vi "SV Change notification event builder.vi"(8 "error in (no error)":errorcluster, 11 "Guardian in":refnum<class "Guardian.lvclass">) -> (0 "error out":errorcluster, 3 "shared variable value change notification":refnum<user-event>)   [LabVIEW 2020, in "TALOS.lvlib" / "Guardian.lvlib" / "Guardian.lvclass"]
uses:
  Guardian.lvclass
  C:/Users/marco/Documents/GitHub_Lab/TALOS/talos/Ancestor/Ancestor/Ancestor.lvclass
  Ancestor/Ancestor/Ancestor.lvclass/Ancestor.ctl
  Classes/Circus Shared Variables/Circus Shared Variables.lvclass/Circus Shared Variables.ctl
  Support VIs/Substitute Error.vi
  Support VIs/Generate Error.vi
  FGV/Error Memory/Get Error Description.vi
  Support VIs/Get PC name.vi
  Support VIs/Get Class Name.vi
  <vilib>/Utility/error.llb/Clear Errors.vi
  FGV/Error Memory/Error Memory Core.vi
  <vilib>/AdvancedString/Delimited String to 1D String Array.vi
  Support VIs/Circus Root Path.vi
  FGV/Error Memory/Error Crt Lvl checker.vi
  FGV/Error Memory/Error Memory Core.vi/40c8088d-b597-4017-91af-faa98e00292e.vi
  FGV/Error Memory/Error Memory Core.vi/d4a3ab98-063c-4e44-b43d-fbdcfe6c2be2.vi
  Support VIs/Global Constants.vi
  Support VIs/Global Memory.vi
  <vilib>/Utility/LVClass/Get LV Class Name.vi
  Support VIs/Is in Packed Library.vi
  Support VIs/TALOS Root path.vi
  Support VIs/Read CSV worksheet.vi
  <vilib>/Utility/error.llb/General Error Handler.vi
  Support VIs/Error Log.vi
  Ancestor/Ancestor/Ancestor.lvclass
  <vilib>/Comparison/Equal/Equal Functor/Equal Functor.lvclass
  <vilib>/lvdsc/NI_DSC.lvlib
  TALOS.lvlib
  Classes/Circus Shared Variables/Circus Shared Variables.lvclass
  Classes/Guardian List/Guardian List.lvclass
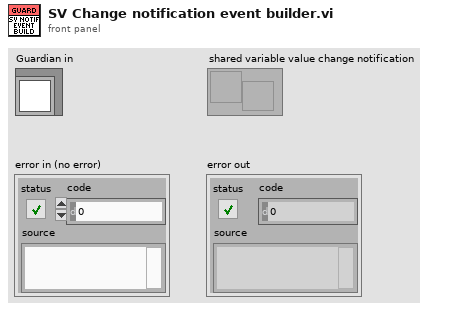
[diagram p1: front panel]
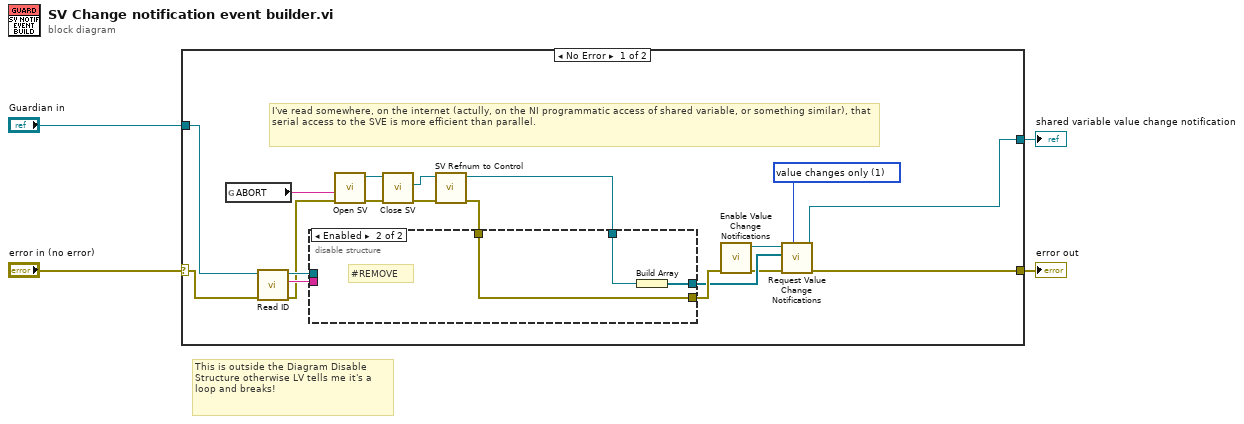
[diagram p0: block diagram]
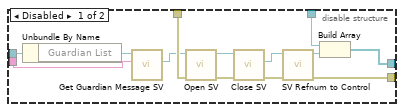
[diagram p2: hidden frame]
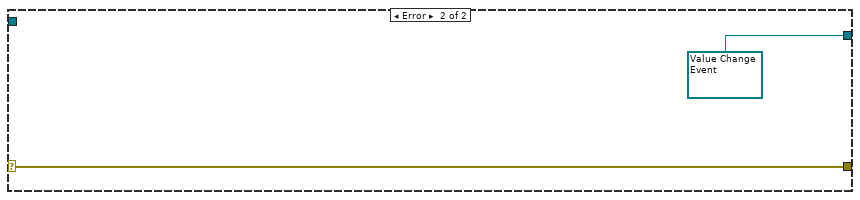
[diagram p3: hidden frame]
diagram:
  # "This is outside the Diagram Disable Structure otherwise LV tells me it's a loop and breaks!"
  n1 = case shown="No Error" "error in (no error)" {
    selector: "error in (no error)" -> [w6 w41]
    tunnel: "Guardian in" -> [w20 _]
    tunnel: [w17 refnum<user-event> refnum ("shared variable value change notification")] -> w2
    tunnel: [w10 w41] -> w1
    frame No Error {
      w18 = u16 1 items=["all changes", "value changes only"] ("request changes (all changes)")
      # "I've read somewhere, on the internet (actully, on the NI programmatic access of shared variable, or something similar), that serial access to the SVE is more efficient than parallel."
      n2 = global read "Global Constants.vi" "ABORT"() -> (w23:string)
      n3 = call "Read ID.vi"("error in (no error)"=w6, "Ancestor in"=w20) -> ("error out"=w5:errorcluster, "ID"=w22:string, "Ancestor out"=w19:refnum<class "Guardian.lvclass">)  [unwired: 7 in]
      n4 = call "Open SV.vi"("error in (no error)"=w5, "SV Name"=w23) -> ("error out"=w12:errorcluster, "AEgIS Shared Variables out"=w11:refnum<class "Circus Shared Variables.lvclass">)  [unwired: 8 in]
      n5 = call "Close SV.vi"("error in (no error)"=w12, "AEgIS Shared Variables in"=w11) -> ("error out"=w15:errorcluster, "SV"=w13:refnum<k21>)  [unwired: 7 in, 1 out]
      n6 = call "SV Refnum to Control.vi"("error in (no error)"=w15, "shared variable refnum in"=w13) -> ("error out"=w21:errorcluster, "Shared Variable Control Out"=w14:refnum<k21>)  [unwired: 8 in]
      n7 = disable-structure shown="Enabled" {
        disable-tunnel: w22 -> [w36 _]
        disable-tunnel: w21 -> [w35 w39]
        disable-tunnel: w19 -> [w29 _]
        disable-tunnel: [w26 w39] -> w16
        disable-tunnel: w14 -> [w25 w38]
        disable-tunnel: [w24 w37] -> w9
        frame Disabled {
          n8 = Unbundle By Name(w29) -> ("Guardian List"=w28:refnum<class "Guardian List.lvclass">)
          n9 = call-dynamic "Get Guardian Message SV.vi"("ID"=w36, "Guardian List in"=w28) -> ("Guardian Message"=w31:refnum<class "Circus Shared Variables.lvclass">)  [unwired: 7 in, 2 out]
          n10 = call "Open SV.vi"("error in (no error)"=w35, "AEgIS Shared Variables in"=w31) -> ("error out"=w32:errorcluster, "AEgIS Shared Variables out"=w30:refnum<class "Circus Shared Variables.lvclass">)  [unwired: 8 in]
          n11 = call "Close SV.vi"("error in (no error)"=w32, "AEgIS Shared Variables in"=w30) -> ("error out"=w33:errorcluster, "SV"=w34:refnum<k21>)  [unwired: 7 in, 1 out]
          n12 = call "SV Refnum to Control.vi"("error in (no error)"=w33, "shared variable refnum in"=w34) -> ("error out"=w26:errorcluster, "Shared Variable Control Out"=w27:refnum<k21>)  [unwired: 8 in]
          n13 = Build Array(w25, w27) -> (w24:refnum<k21>[])
        }
        frame Enabled {
          # "#REMOVE"
          n14 = Build Array(w38) -> (w37:refnum<k21>[])
        }
      }
      n15 = call <vilib>:"Enable Value Change Notifications.vi"("error in (no error)"=w16) -> ("error out"=w8:errorcluster, "shared variable value change notification"=w7:refnum<user-event>)  [unwired: 9 in]
      n16 = call <vilib>:"Request Value Change Notifications.vi"("request changes (all changes)"=w18, "error in (no error)"=w8, "shared variables"=w9, "notification refnum"=w7) -> ("error out"=w10:errorcluster, "shared variable value change notification"=w17:refnum<user-event>)  [unwired: 5 in, 1 out]
    }
    frame Error {
    }
  }
  "shared variable value change notification" <- w2
  "error out" <- w1
